vi "Stop Core.vi"(10 "final error code":i32, 11 "CS++DMM in":refnum<class "CS++DMM.lvclass">) -> (3 "CS++DMM out":refnum<class "CS++DMM.lvclass">)   [LabVIEW 2013, in "CS++DMM.lvlib" / "CS++DMM.lvclass"]
doc: "(<B>Filename</B>: Actor Framework.lvlib:Actor.lvclass:Stop Core.vi)\n\nDefines what the actor does before it stops. Use the <B>final error code</B> input to determine whether the actor shut down in response to an error.\n\nBy default, this method does nothing. A descendant class may override it to define behavior, such as shutting down any processes the actor initiated in its override of the Actor Core method."
uses:
  CS++DMM.lvclass
  CSPP_Core/Actors/CS++DeviceActor/CS++DeviceActor.lvclass
  CSPP_Core/Classes/CS++ProcessVariables/PVConnection/PVConnection.lvclass
  <vilib>/ActorFramework/Time-Delayed Send Message/Time-Delay Override Options.ctl
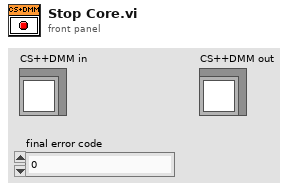
[diagram p1: front panel]
types:
  T1 = typedef "Time-Delay Override Options.ctl" = enum16{"Send next copy now", "Skip next scheduled copy", "Send next copy now and stop all further copies", "Stop all further copies"}
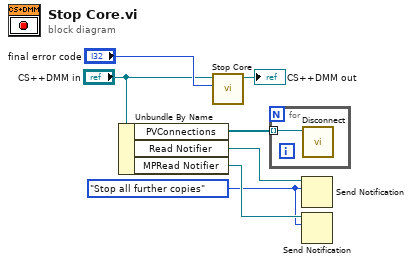
[diagram p0: block diagram]
diagram:
  w2 = Time-Delay_Override_Options."Stop all further copies" ("notification")
  n1 = Unbundle By Name("CS++DMM in") -> ("PVConnections"=w1:refnum<class "PVConnection.lvclass">[], "Read Notifier"=w4:refnum<notifier>, "MPRead Notifier"=w3:refnum<notifier>)
  n2 = call-parent "Stop Core.vi"("final error code"="final error code", "CS++DeviceActor in"="CS++DMM in") -> ("CS++DeviceActor out"=→"CS++DMM out":refnum<class "CS++DMM.lvclass">)  [unwired: 9 in]
  n3 = for {
    tunnel: w1 -> [w8] mode=indexing
    n4 = call-dynamic "Disconnect.vi"("PVConnection in"=w8) -> ()  [unwired: 9 in, 2 out]
  }
  n5 = Send Notification(notification=w2, notifier=w4) -> ()  [unwired: 1 in, 2 out]
  n6 = Send Notification(notification=w2, notifier=w3) -> ()  [unwired: 1 in, 2 out]
